vi "getfluxpoint.vi"(5 "flux":dbl, 11 "Plot":cluster{cluster{dbl, "icn":dbl}[]}) -> (2 "phase0":dbl, 3 "actual flux":dbl)   [LabVIEW 2023]
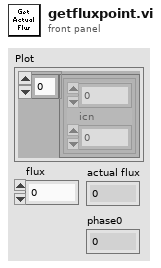
[diagram p1: front panel]
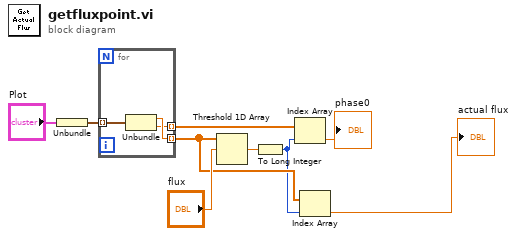
[diagram p0: block diagram]
diagram:
  n1 = Unbundle("Plot") -> (w8:cluster{dbl, "icn":dbl}[])
  n2 = for {
    tunnel: w8 -> [w12] mode=indexing
    tunnel: [w11] -> w4 mode=indexing
    tunnel: [w10] -> w5 mode=indexing
    n3 = Unbundle(w12) -> (w11:dbl, "icn"=w10:dbl)
  }
  n4 = Threshold 1D Array(2:"flux", 3:w4) -> (0:w6:dbl)  [unwired: 1 in]
  n5 = To Long Integer(number=w6) -> (32bit integer=w3:i32)
  n6 = Index Array(array=w5, index=w3) -> (element=→"phase0":dbl)
  n7 = Index Array(array=w4, index=w3) -> (element=→"actual flux":dbl)
